vi "Supply_ReadCurrent.vi"(8 "error in (no error)":errorcluster, 11 "KE237 in":refnum<class "KE237.lvclass">) -> (0 "error out":errorcluster, 2 "Current in nA":dbl format="%#.6g", 3 "KE237 out":refnum<class "KE237.lvclass">)   [LabVIEW 2018, in "KE237.lvclass"]
uses:
  KE237.lvclass
  <vilib>/regexp/Match Regular Expression.xnode
panel:
  out "compliance letter":string
  out "Status string":string
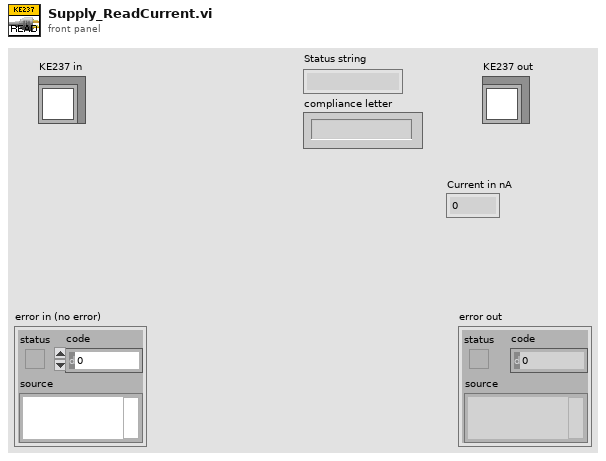
[diagram p1: front panel]
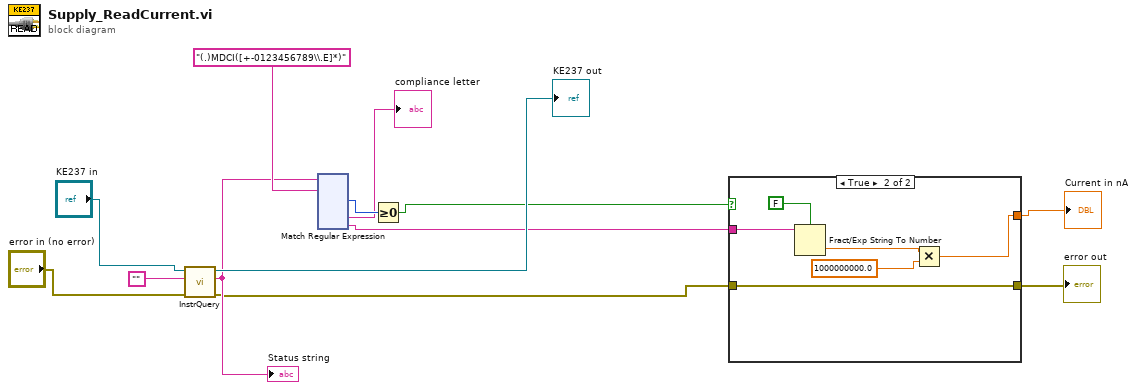
[diagram p0: block diagram]
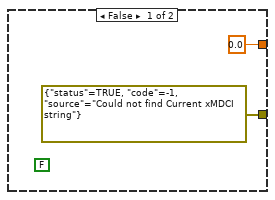
[diagram p2: hidden frame]
diagram:
  n1 = call-dynamic "InstrQuery.vi"("error in (no error)"="error in (no error)", "Command string"="", "InstControl in"="KE237 in") -> ("error out"=w3:errorcluster, "Instrument response"=w8:string, "InstControl out"=→"KE237 out":refnum<class "KE237.lvclass">)  [unwired: 6 in]
  "Status string" <- w8
  n2 = xnode "Match Regular Expression"("input string"=w8, "regular expression"="(.)MDCI([+-0123456789\\.E]*)") -> ("offset past match"=w7:i32, "submatch 1"=→"compliance letter":string, "submatch 2"=w4:string)  [unwired: 4 in, 4 out]
  n3 = Greater Or Equal To 0?(x=w7) -> (x >= 0?=w2:bool)
  n4 = case shown="True" w2 {
    tunnel: [errorcluster {"status"=TRUE, "code"=-1, "source"="Could not find Current xMDCI string"} ("error out") w16] -> w5
    tunnel: w3 -> [_ w16]
    tunnel: w4 -> [_ w21]
    tunnel: [0.0 w17] -> w1
    frame False {
      (unwired) FALSE ("Compliance exceeded?")
    }
    frame True {
      n5 = Fract/Exp String To Number(use system decimal point (T)=FALSE, string=w21) -> (number=w19:dbl)  [unwired: 2 in, 1 out]
      n6 = Multiply(x=w19, y=1000000000.0 ("number")) -> (x*y=w17:dbl)
    }
  }
  "error out" <- w5
  "Current in nA" <- w1
